vi "niRFUtil FWK Find Rational Divisors.vi"(0 "Number":i32=19000, 5 "Maximum Divisor":i32=1000, 7 "Minimum Divisor":i32=10, 11 "error in (no error)":errorcluster) -> (4 "Divisors":i32[](array[numeric]), 15 "error out":errorcluster)   [LabVIEW 2015, in "niRFUtil.lvlib"]
uses:
  niRFUtil.lvlib
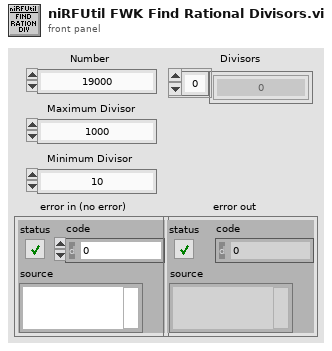
[diagram p1: front panel]
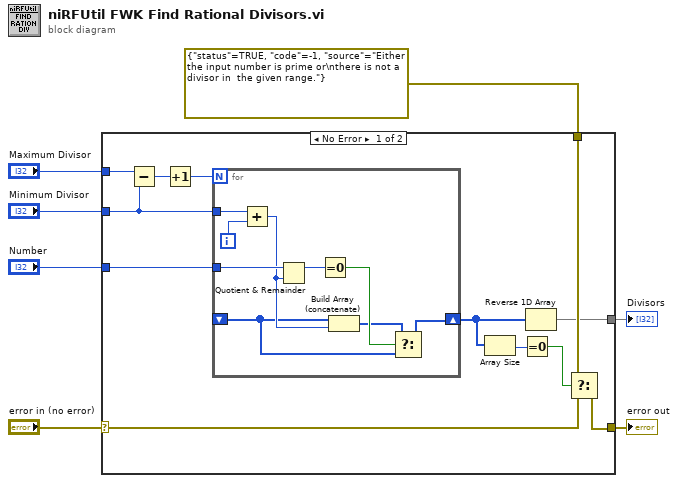
[diagram p0: block diagram]
diagram:
  n1 = case shown="No Error" "error in (no error)" {
    selector: "error in (no error)" -> [w12 w29]
    tunnel: [w11 w29] -> w6
    tunnel: "Maximum Divisor" -> [w19 _]
    tunnel: "Minimum Divisor" -> [w17 _]
    tunnel: "Number" -> [w16 _]
    tunnel: [w8 _] -> w2
    tunnel: errorcluster {"status"=TRUE, "code"=-1, "source"="Either the input number is prime or\nthere is not a divisor in  the given range."} ("t") -> [w10 _]
    frame No Error {
      n2 = Subtract(x=w19, y=w17) -> (x-y=w18:i32)
      n3 = Increment(x=w18) -> (x+1=w9:i32)
      n4 = for {
        N: w9 -> [_]
        shift-right: [w22] -> w15
        shift-left: _ -> [w20]
        tunnel: w17 -> [w27]
        tunnel: w16 -> [w23]
        i -> [w28]
        n5 = Add(x=w27, y=w28) -> (x+y=w21:i32)
        n6 = Quotient & Remainder(x=w23, y=w21) -> (x-y*floor(x/y)=w26:i32)  [unwired: 1 out]
        n7 = Equal To 0?(x=w26) -> (x = 0?=w25:bool)
        n8 = Build Array (concatenate)(w20, w21) -> (w24:i32[])
        n9 = Select(t=w24, s=w25, f=w20) -> (s? t:f=w22:i32[])
      }
      n10 = Array Size(array=w15) -> (size(s)=w14:i32)
      n11 = Equal To 0?(x=w14) -> (x = 0?=w13:bool)
      n12 = Reverse 1D Array(array=w15) -> (reversed array=w8:i32[])
      n13 = Select(t=w10, s=w13, f=w12) -> (s? t:f=w11:errorcluster)
    }
    frame Error {
    }
  }
  "Divisors" <- w2
  "error out" <- w6
